vi "Get Group From Memory.vi"(8 "error in (no error)":errorcluster, 10 "Group":string, 11 "(Re)initialize? (F)":bool) -> (0 "error out":errorcluster, 3 "CVT File Data":T1)   [LabVIEW 2016, in "CVT.lvlib" / "Current Value Table.lvlib"]
doc: "This VI fetches all tags currently in the engine and generates a tag list similar to the function used to initialize the CVT. This is actually a functional global variable which stores all the tags and their indices. When the function is called the first time, or if the (re)initialize boolean is set, it will retrieve all tags from the CVT along with their indices. This process takes approximately 200 ms for 1000 tags on the cRIO 9076. Subsequent calls are much faster, as they simply read the required data from the CVT memblock."
uses:
  <vilib>/NI/Current Value Table/Current Value Table.lvlib
  <vilib>/NI/Current Value Table/Type Defs/File Format.ctl
  <vilib>/NI/Current Value Table/Type Defs/Single Tag.ctl
  <vilib>/NI/Current Value Table/Type Defs/Data Types.ctl
  <vilib>/NI/Current Value Table/Type Defs/Tag Grouping set.ctl
  <vilib>/NI/Current Value Table/FGVs/Tag Memory Methods.ctl
  <vilib>/NI/Current Value Table/FGVs/Group Memory Methods.ctl
  <vilib>/NI/Current Value Table/Scan tag to value.vi
  <vilib>/NI/Current Value Table/Data To ASCII String.vi
  <vilib>/NI/Current Value Table/DataTypes/Double_Data To ASCII String.vi
  <vilib>/NI/Current Value Table/Read Index.vi
  <vilib>/NI/Current Value Table/DataTypes/Double_Read Index.vi
  <vilib>/NI/Current Value Table/DataTypes/Array of String_Data To ASCII String.vi
  <vilib>/NI/Current Value Table/DataTypes/Array of String_Read Index.vi
  <vilib>/NI/Current Value Table/DataTypes/Array of Boolean_Data To ASCII String.vi
  <vilib>/NI/Current Value Table/DataTypes/Array of Boolean_Read Index.vi
  <vilib>/NI/Current Value Table/DataTypes/Array of Single_Data To ASCII String.vi
  <vilib>/NI/Current Value Table/DataTypes/Array of Single_Read Index.vi
  <vilib>/NI/Current Value Table/DataTypes/Array of Double_Data To ASCII String.vi
  <vilib>/NI/Current Value Table/DataTypes/Array of Double_Read Index.vi
  <vilib>/NI/Current Value Table/DataTypes/Array of I8_Data To ASCII String.vi
  <vilib>/NI/Current Value Table/DataTypes/Array of I8_Read Index.vi
  <vilib>/NI/Current Value Table/DataTypes/Array of I16_Data To ASCII String.vi
  <vilib>/NI/Current Value Table/DataTypes/Array of I16_Read Index.vi
  <vilib>/NI/Current Value Table/DataTypes/Array of I32_Data To ASCII String.vi
  <vilib>/NI/Current Value Table/DataTypes/Array of I32_Read Index.vi
  <vilib>/NI/Current Value Table/DataTypes/Array of I64_Data To ASCII String.vi
  <vilib>/NI/Current Value Table/DataTypes/Array of I64_Read Index.vi
  <vilib>/NI/Current Value Table/DataTypes/Array of U64_Data To ASCII String.vi
  <vilib>/NI/Current Value Table/DataTypes/Array of U64_Read Index.vi
  <vilib>/NI/Current Value Table/DataTypes/Array of U32_Data To ASCII String.vi
  <vilib>/NI/Current Value Table/DataTypes/Array of U32_Read Index.vi
  <vilib>/NI/Current Value Table/DataTypes/Array of U16_Data To ASCII String.vi
  <vilib>/NI/Current Value Table/DataTypes/Array of U16_Read Index.vi
  <vilib>/NI/Current Value Table/DataTypes/Array of U8_Data To ASCII String.vi
  <vilib>/NI/Current Value Table/DataTypes/Array of U8_Read Index.vi
  <vilib>/NI/Current Value Table/DataTypes/Boolean_Data To ASCII String.vi
  <vilib>/NI/Current Value Table/DataTypes/Boolean_Read Index.vi
  <vilib>/NI/Current Value Table/DataTypes/String_Data To ASCII String.vi
  <vilib>/NI/Current Value Table/DataTypes/String_Read Index.vi
  <vilib>/NI/Current Value Table/DataTypes/U8_Data To ASCII String.vi
  <vilib>/NI/Current Value Table/DataTypes/U8_Read Index.vi
  <vilib>/NI/Current Value Table/DataTypes/U16_Data To ASCII String.vi
  <vilib>/NI/Current Value Table/DataTypes/U16_Read Index.vi
  <vilib>/NI/Current Value Table/DataTypes/U32_Data To ASCII String.vi
  <vilib>/NI/Current Value Table/DataTypes/U32_Read Index.vi
  <vilib>/NI/Current Value Table/DataTypes/U64_Data To ASCII String.vi
  <vilib>/NI/Current Value Table/DataTypes/U64_Read Index.vi
  <vilib>/NI/Current Value Table/DataTypes/I8_Data To ASCII String.vi
  <vilib>/NI/Current Value Table/DataTypes/I8_Read Index.vi
  <vilib>/NI/Current Value Table/DataTypes/I16_Data To ASCII String.vi
  <vilib>/NI/Current Value Table/DataTypes/I16_Read Index.vi
  <vilib>/NI/Current Value Table/DataTypes/I32_Data To ASCII String.vi
  <vilib>/NI/Current Value Table/DataTypes/I32_Read Index.vi
  <vilib>/NI/Current Value Table/DataTypes/I64_Data To ASCII String.vi
  <vilib>/NI/Current Value Table/DataTypes/I64_Read Index.vi
  <vilib>/NI/Current Value Table/DataTypes/Single_Data To ASCII String.vi
  <vilib>/NI/Current Value Table/DataTypes/Single_Read Index.vi
  <vilib>/NI/Current Value Table/Memory Block.vi
  <vilib>/NI/Current Value Table/DataTypes/Single_Memory Block.vi
  <vilib>/NI/Current Value Table/DataTypes/I64_Memory Block.vi
  <vilib>/NI/Current Value Table/DataTypes/I32_Memory Block.vi
  <vilib>/NI/Current Value Table/DataTypes/I16_Memory Block.vi
  <vilib>/NI/Current Value Table/DataTypes/I8_Memory Block.vi
  <vilib>/NI/Current Value Table/DataTypes/U64_Memory Block.vi
  <vilib>/NI/Current Value Table/DataTypes/U32_Memory Block.vi
  <vilib>/NI/Current Value Table/DataTypes/U16_Memory Block.vi
  <vilib>/NI/Current Value Table/DataTypes/U8_Memory Block.vi
  <vilib>/NI/Current Value Table/DataTypes/String_Memory Block.vi
  <vilib>/NI/Current Value Table/DataTypes/Boolean_Memory Block.vi
  <vilib>/NI/Current Value Table/DataTypes/Array of U8_Memory Block.vi
  <vilib>/NI/Current Value Table/DataTypes/Array of U16_Memory Block.vi
  <vilib>/NI/Current Value Table/DataTypes/Array of U32_Memory Block.vi
  <vilib>/NI/Current Value Table/DataTypes/Array of U64_Memory Block.vi
  <vilib>/NI/Current Value Table/DataTypes/Array of I64_Memory Block.vi
  <vilib>/NI/Current Value Table/DataTypes/Array of I32_Memory Block.vi
  <vilib>/NI/Current Value Table/DataTypes/Array of I16_Memory Block.vi
  <vilib>/NI/Current Value Table/DataTypes/Array of I8_Memory Block.vi
  <vilib>/NI/Current Value Table/DataTypes/Array of Double_Memory Block.vi
  <vilib>/NI/Current Value Table/DataTypes/Array of Single_Memory Block.vi
  <vilib>/NI/Current Value Table/DataTypes/Array of Boolean_Memory Block.vi
  <vilib>/NI/Current Value Table/DataTypes/Array of String_Memory Block.vi
  <vilib>/NI/Current Value Table/DataTypes/Double_Memory Block.vi
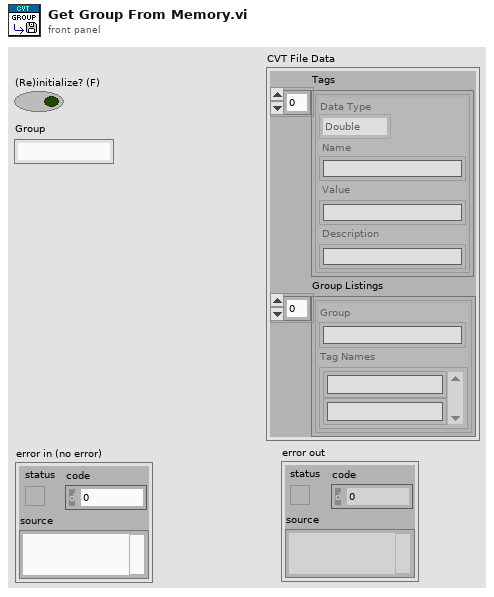
[diagram p1: front panel]
types:
  T1 = typedef "CVT.lvlib/Current Value Table.lvlib/File Format.ctl" = cluster{"Tags":T2[], "Group Listings":T4[]}
  T2 = typedef "CVT.lvlib/Current Value Table.lvlib/Single Tag.ctl" = cluster{"Data Type":T3, "Name":string, "Value":string, "Description":string}
  T3 = typedef "CVT.lvlib/Current Value Table.lvlib/Data Types.ctl" = enum16{"Double", "Single", "I64", "I32", "I16", "I8", "U64", "U32", "U16", "U8", "String", "Boolean", "Array of U8", "Array of U16", "Array of U32", "Array of U64", "Array of I64", "Array of I32", "Array of I16", "Array of I8", "Array of Double", "Array of Single", "Array of Boolean", "Array of String"}
  T4 = typedef "CVT.lvlib/Current Value Table.lvlib/Tag Grouping set.ctl" = cluster{"Group":string, "Tag Names":string[]}
  T5 = typedef "CVT.lvlib/Current Value Table.lvlib/Tag in Memory.ctl" = cluster{"Index":i32, "Tag":T2}
  T6 = typedef "CVT.lvlib/Current Value Table.lvlib/Group Memory Methods.ctl" = enum16{"Clear", "Read Indices in Group", "List Groups", "List Tags by Type", "List Tags", "Delete Group", "Check Group Existence", "Create Group"}
  T7 = typedef "CVT.lvlib/Current Value Table.lvlib/Tag Memory Methods.ctl" = enum16{"Clear", "Read Tag Index", "Read Tag Indices", "Generate Group", "Add Tag", "Overwrite Tag", "Read Description", "Get Stored Tags"}
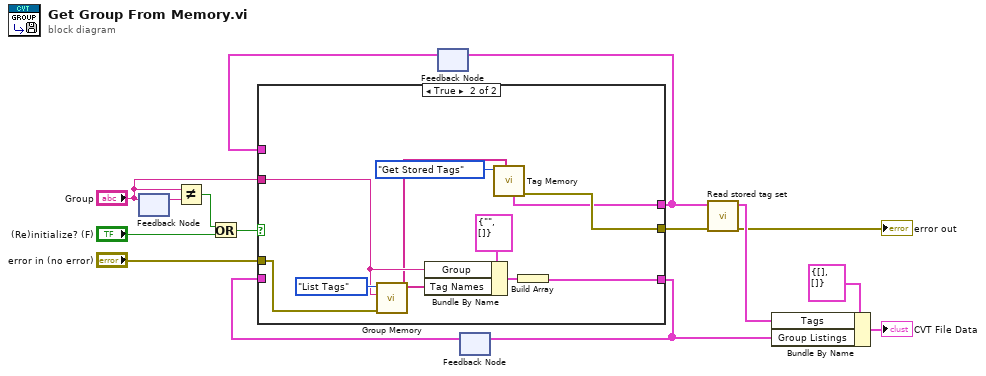
[diagram p0: block diagram]
diagram:
  n1 = feedback #1() -> (w7:string)  [unwired: 1 in]
  n2 = feedback-in #1("Group") -> ()
  n3 = Not Equal?(x="Group", y=w7) -> (x != y?=w8:bool)
  n4 = Or(x=w8, y="(Re)initialize? (F)") -> (x .or. y?=w10:bool)
  n5 = feedback #2() -> (w15:T5[])  [unwired: 1 in]
  n6 = feedback #3() -> (w14:T4[])  [unwired: 1 in]
  n7 = case shown="True" w10 {
    tunnel: "error in (no error)" -> [w18 w22]
    tunnel: [w18 w28] -> w4
    tunnel: [w17 w21] -> w3
    tunnel: w15 -> [w17 _]
    tunnel: [w16 w23] -> w12
    tunnel: w14 -> [w16 _]
    tunnel: "Group" -> [_ w20]
    frame False {
    }
    frame True {
      n8 = call <vilib>:"Group Memory.vi"("error in (no error)"=w22, "Group"=w20, "Method"=Group_Memory_Methods."List Tags") -> ("Tags/Groups Out"=w19:string[])  [unwired: 5 in, 3 out]
      n9 = Bundle By Name(cluster=T4 {"Group"="", "Tag Names"=[]} ("Tag Grouping"), "Group"=w20, "Tag Names"=w19) -> (w26:T4)
      n10 = call <vilib>:"Tag Memory.vi"("Tags"=w19, "Method"=Tag_Memory_Methods."Get Stored Tags") -> ("error out"=w28:errorcluster, "Stored Tags"=w21:T5[])  [unwired: 4 in, 4 out]
      n11 = Build Array(w26) -> (w23:T4[])
    }
  }
  n12 = feedback-in #2(w3) -> ()
  n13 = feedback-in #3(w12) -> ()
  n14 = call <vilib>:"Read stored tag set.vi"("error in (no error)"=w4, "stored tags"=w3) -> ("error out"=→"error out":errorcluster, "Tags"=w2:T2[])  [unwired: 8 in]
  n15 = Bundle By Name(cluster=T1 {"Tags"=[], "Group Listings"=[]} ("File Format"), "Tags"=w2, "Group Listings"=w12) -> (→"CVT File Data":T1)
